vi "ElevatorDashReadOuterNetwork.vi"() -> (0 "OuterOnTarget":bool, 1 "OuterMotorOutput":dbl, 2 "OuterPositionHeight":dbl, 3 "OuterPosDemandHeight":dbl, 4 "OuterHighLimitSwitch":bool, 6 "OuterLowLimitSwitch":bool)   [LabVIEW 2023]
uses:
  <vilib>/Rock Robotics/Network Tables/NT Read Boolean.vi
  <vilib>/Rock Robotics/Network Tables/NT Read Number.vi
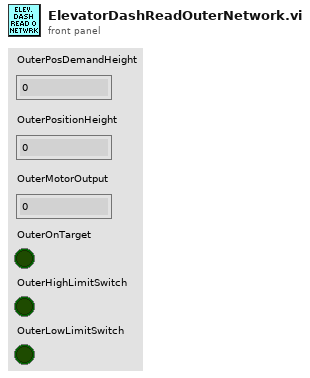
[diagram p1: front panel]
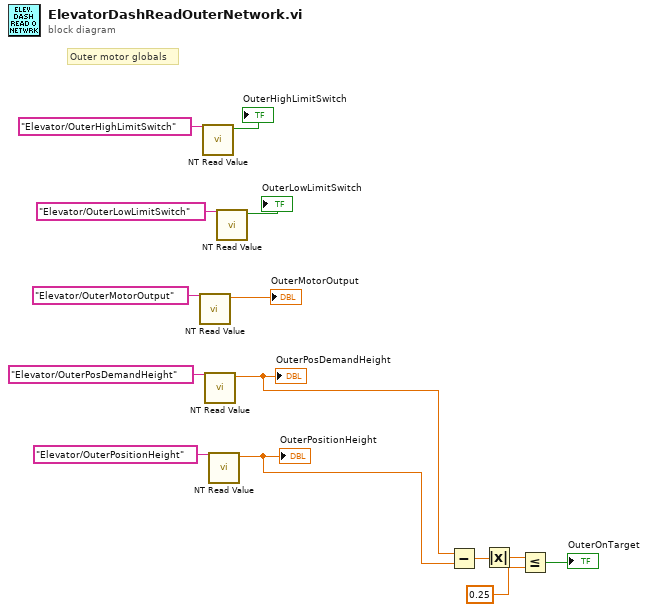
[diagram p0: block diagram]
diagram:
  # "Outer motor globals"
  n1 = call-poly <vilib>:"NT Read Value.vi"("name"="Elevator/OuterMotorOutput") -> ("value"=→"OuterMotorOutput":dbl)  [unwired: 8 in, 2 out]
  n2 = call-poly <vilib>:"NT Read Value.vi"("name"="Elevator/OuterHighLimitSwitch") -> ("value"=→"OuterHighLimitSwitch":bool)  [unwired: 8 in, 2 out]
  n3 = call-poly <vilib>:"NT Read Value.vi"("name"="Elevator/OuterPosDemandHeight") -> ("value"=w2:dbl)  [unwired: 8 in, 2 out]
  "OuterPosDemandHeight" <- w2
  n4 = call-poly <vilib>:"NT Read Value.vi"("name"="Elevator/OuterPositionHeight") -> ("value"=w1:dbl)  [unwired: 8 in, 2 out]
  "OuterPositionHeight" <- w1
  n5 = call-poly <vilib>:"NT Read Value.vi"("name"="Elevator/OuterLowLimitSwitch") -> ("value"=→"OuterLowLimitSwitch":bool)  [unwired: 8 in, 2 out]
  n6 = Subtract(x=w2, y=w1) -> (x-y=w9:dbl)
  n7 = Absolute Value(x=w9) -> (abs(x)=w8:dbl)
  n8 = Less Or Equal?(x=w8, y=0.25) -> (x <= y?=→"OuterOnTarget":bool)
